vi "Deinitialize.vi"(8 "error in (no error)":errorcluster, 11 "IP Connection in":refnum<class "IP Connection.lvclass">) -> (0 "error out":errorcluster)   [LabVIEW 2011, in "Tinkerforge.lvlib" / "IP Connection.lvclass"]
doc: "This VI deinitializes the <B>IP Connection</B> class object and collects the called communication worker VI and disconnects from the Brickd."
uses:
  IP Connection.lvclass
  IP Connection.lvclass/IP Connection.ctl
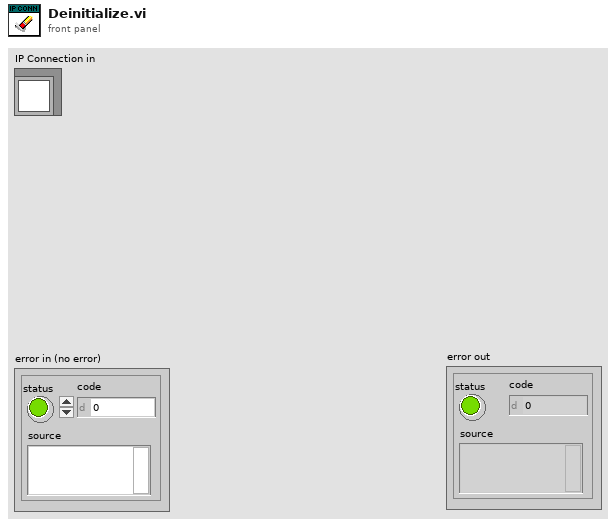
[diagram p1: front panel]
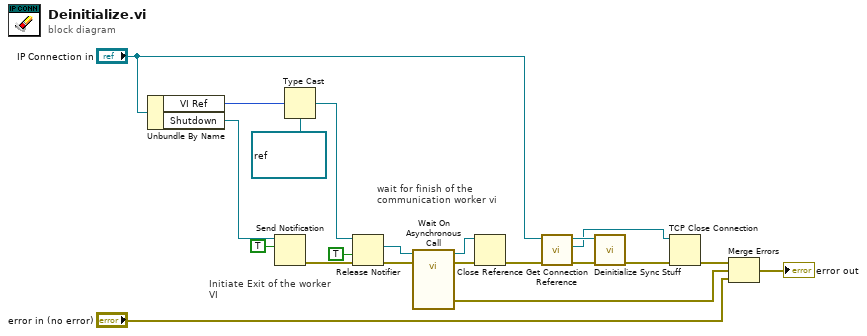
[diagram p0: block diagram]
diagram:
  # "Initiate Exit of the worker\nVI"
  # "wait for finish of the\ncommunication worker vi"
  n1 = Unbundle By Name("IP Connection in") -> ("VI Ref"=w21:u32, "Shutdown"=w7:refnum<notifier>)
  n2 = Send Notification(notification=TRUE, notifier=w7) -> (error out=w8:errorcluster)  [unwired: 1 in, 1 out]
  n3 = Type Cast(type=refnum<notifier> refnum ("notifier out"), x=w21) -> (*(type *) &x=w18:refnum<notifier>)
  n4 = Release Notifier(notifier=w18, force destroy? (F)=TRUE, error in (no error)=w8) -> (last notification=w17:refnum<vi>, error out=w19:errorcluster)  [unwired: 1 out]
  n5 = call-by-ref "Wait On Asynchronous Call"(reference=w17, error in=w19) -> (reference out=w14:refnum<vi>, error out=w15:errorcluster, 0:"error out"=w10:errorcluster)  [unwired: 10 in, 1 out]
  n6 = Close Reference(reference=w14, error in (no error)=w15) -> (error out=w5:errorcluster)
  n7 = call "Get Connection Reference.vi"("error in (no error)"=w5, "IP Connection in"="IP Connection in") -> ("error out"=w2:errorcluster, "TCP Network Connection"=w1:refnum<k5>, "IP Connection out"=w3:refnum<class "IP Connection.lvclass">)  [unwired: 7 in]
  n8 = call "Deinitialize Sync Stuff.vi"("error in (no error)"=w2, "IP Connection in"=w3) -> ("error out"=w12:errorcluster)  [unwired: 8 in, 1 out]
  n9 = TCP Close Connection(connection ID=w1, error in (no error)=w12) -> (error out=w11:errorcluster)  [unwired: 1 in, 1 out]
  n10 = Merge Errors(w11, w10, "error in (no error)") -> (→"error out":errorcluster)
